vi "Get Device Information.vi"(11 "SOL Camera in":refnum<class "PL SOL Instruments Camera.lvclass">) -> (1 "camera information":T1 {"sensor type" items=["unknown"=0, "S9840"=1, "S7017-1007"=10, "S7017-1008"=11, "S7030-0908"=20, "S7030-1006"=21, "S7030-1008"=22, "S7031-1006"=30, "S7031-1007"=31, "S7031-1008"=32, "S7170-0909"=40, "S7171-0909"=41, "S7172-0909"=42, "S8378-1024Q"=50, "S8667-1010"=51, "S9737-01"=60, "S9970-1007"=70, "S10141-1109"=80, "S10142-1107"=90, "S10142-1108"=91, "S10142-1109"=92, "G9201-256S"=100, "G9202-512S"=101, "G9203-256S"=102, "G9204-512S"=103, "G9208-256W"=104, "I5-A1300-M2"=110, "I5-A1300-C2"=111, "LUPA-4000M"=200]; "cooling"."type" items=["no sensors", "3 sensors", "1 sensor"]}, 2 "controller information":T2, 3 "SOL Camera out":refnum<class "PL SOL Instruments Camera.lvclass">)   [LabVIEW 2015, in "PL SOL Instruments Camera.lvclass"]
doc: "Returns controller and camera information."
uses:
  PL SOL Instruments Camera.lvclass
  PL SOL Instruments Camera.lvclass/PL SOL Instruments Camera.ctl
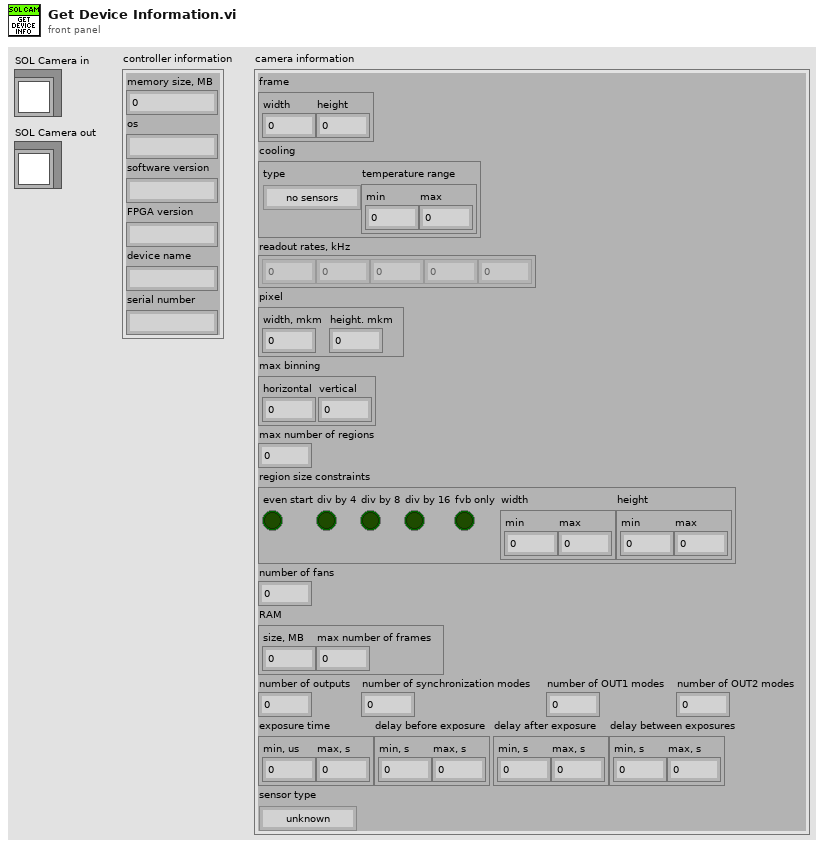
[diagram p1: front panel]
types:
  T1 = cluster{"frame":cluster{"width":u16, "height":u16}, "cooling":cluster{"type":u16, "temperature range":cluster{"min":i32, "max":i32}}, "readout rates, kHz":i32[], "pixel":cluster{"width, mkm":dbl, "height. mkm":dbl}, "max binning":cluster{"horizontal":u16, "vertical":u16}, "max number of regions":u16, "region size constraints":cluster{"even start":bool, "div by 4":bool, "div by 8":bool, "div by 16":bool, "fvb only":bool, "width":cluster{"min":u16, "max":u16}, "height":cluster{"min":u16, "max":u16}}, "number of fans":u16, "RAM":cluster{"size, MB":u16, "max number of frames":u32}, "number of outputs":u16, "number of synchronization modes":u16, "number of OUT1 modes":u16, "number of OUT2 modes":u16, "exposure time":cluster{"min, us":dbl, "max, s":dbl}, "delay before exposure":cluster{"min, s":dbl, "max, s":dbl}, "delay after exposure":cluster{"min, s":dbl, "max, s":dbl}, "delay between exposures":cluster{"min, s":dbl, "max, s":dbl}, "sensor type":u16}
  T2 = cluster{"memory size, MB":i32, "os":string, "software version":string, "FPGA version":string, "device name":string, "serial number":string}
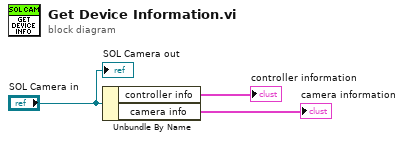
[diagram p0: block diagram]
diagram:
  n1 = Unbundle By Name("SOL Camera in") -> ("controller info"=→"controller information":T2, "camera info"=→"camera information":T1)
  "SOL Camera out" <- "SOL Camera in"
